vi "Array Weighted Average.vi"(4 "Reject NaN (T)":bool=TRUE, 6 "Reject Negative Weights (F)":bool, 8 "Error In":errorcluster, 9 "Weight Array":dbl[](array[numeric]), 11 "Array":dbl[](array[numeric])) -> (0 "Error Out":errorcluster, 1 "SDV (weighted)":dbl, 2 "SDV (classic)":dbl, 3 "Average Value (weighted)":dbl)   [LabVIEW 2021, in "Arrays.lvlib"]
doc: "Compute a weighted average of the input <B>Array</B> A using the provided <B>Weight Array</B> w:\n\n<A> = (Sum(w_i A_i)_{i = 1....N})/(Sum(w_i)_{i = 1....N})\n\nwhere {A_i}_{i = 1....N} is the input <B>Array</B> and {w_i}_{i = 1....N} is the <B>Weight Array</B>.\n\nIf <B>Reject Negative Weights</B> is true, only the term with w_i >= 0 are retained in both sums.\n\nIf the two arrays have different sizes, the unweighted mean of <B>Array</B> is returned.\n\nTo reject NaN values in the calculation, use the <B>Reject NaN</B> flag."
uses:
  Arrays.lvlib
  <userlib>/_OpenG.lib/array/array.llb/Filter 1D Array with Scalar (DBL)__ogtk.vi
  <vilib>/Analysis/NI_AALBase.lvlib
  <userlib>/_OpenG.lib/array/array.llb/openg_array.lvlib
  <userlib>/_OpenG.lib/array/array.llb/Delete Elements from 1D Array (DBL)__ogtk.vi
panel:
  # "see the AlliGator License on the block diagram (Ctrl+E or Window:Show Block Diagram)"
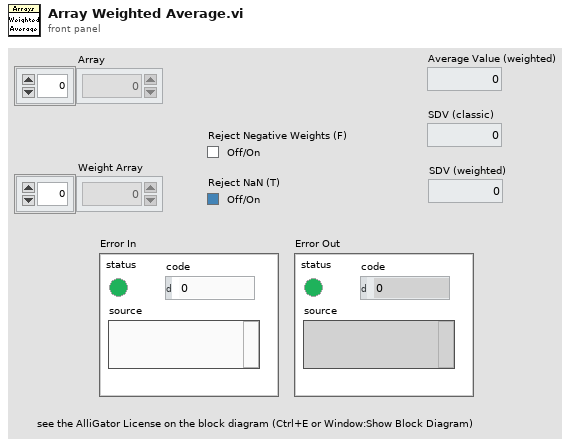
[diagram p1: front panel]
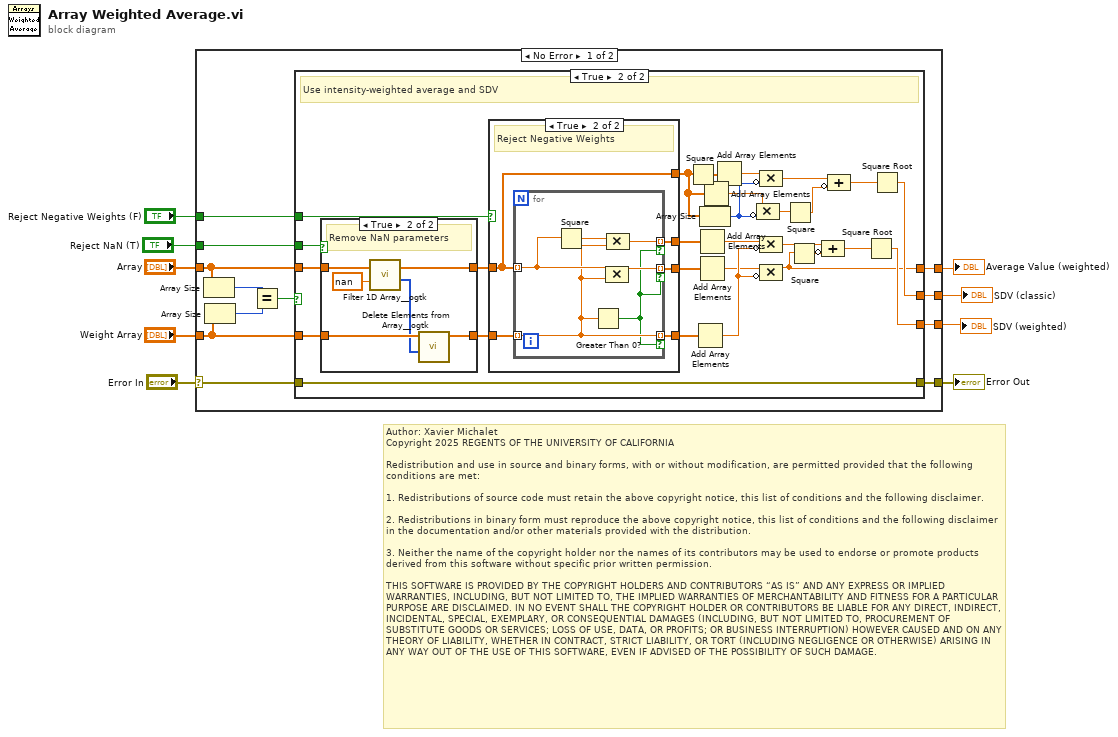
[diagram p0: block diagram]
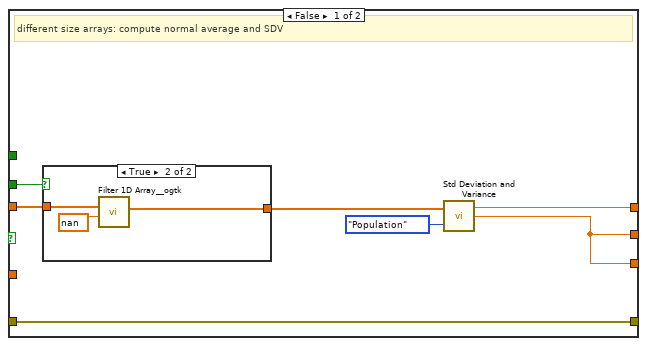
[diagram p2: hidden frame]
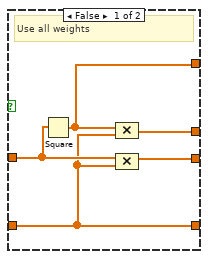
[diagram p5: hidden frame]
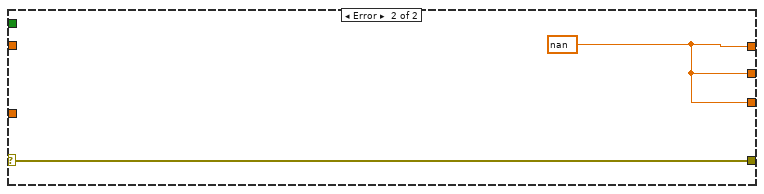
[diagram p6: hidden frame]
diagram:
  # "Author: Xavier Michalet\nCopyright 2025 REGENTS OF THE UNIVERSITY OF CALIFORNIA\n\nRedistribution and use in source and binary forms, with or without modification, are permitted provided that the following conditions are met:\n\n1. Redistributions of source code must retain the above copyright notice, this list of conditions and the following disclaimer.\n\n2. Redistributions in binary form must reproduce the above copyright notice, this list of conditions and the following disclaimer in the documentation and/or other materials provided with the distribution.\n\n3. Neither the name of the copyright holder nor the names of its contributors may be used to endorse or promote products derived from this software without specific prior written permission.\n\nTHIS SOFTWARE IS PROVIDED BY THE COPYRIGHT HOLDERS AND CONTRIBUTORS “AS IS” AND ANY EXPRESS OR IMPLIED WARRANTIES, INCLUDING, BUT NOT LIMITED TO, THE IMPLIED WARRANTIES OF MERCHANTABILITY AND FITNESS FOR A PARTICULAR PURPOSE ARE DISCLAIMED. IN NO EVENT SHALL THE COPYRIGHT HOLDER OR CONTRIBUTORS BE LIABLE FOR ANY DIRECT, INDIRECT, INCIDENTAL, SPECIAL, EXEMPLARY, OR CONSEQUENTIAL DAMAGES (INCLUDING, BUT NOT LIMITED TO, PROCUREMENT OF SUBSTITUTE GOODS OR SERVICES; LOSS OF USE, DATA, OR PROFITS; OR BUSINESS INTERRUPTION) HOWEVER CAUSED AND ON ANY THEORY OF LIABILITY, WHETHER IN CONTRACT, STRICT LIABILITY, OR TORT (INCLUDING NEGLIGENCE OR OTHERWISE) ARISING IN ANY WAY OUT OF THE USE OF THIS SOFTWARE, EVEN IF ADVISED OF THE POSSIBILITY OF SUCH DAMAGE."
  n1 = case shown="No Error" "Error In" {
    selector: "Error In" -> [w13 w86]
    tunnel: "Array" -> [w15 _]
    tunnel: [w19 w85] -> w8
    tunnel: [w12 w86] -> w6
    tunnel: "Weight Array" -> [w14 _]
    tunnel: "Reject Negative Weights (F)" -> [w18 _]
    tunnel: "Reject NaN (T)" -> [w16 _]
    tunnel: [w11 w85] -> w2
    tunnel: [w10 w85] -> w1
    frame No Error {
      n2 = Array Size(array=w15) -> (size(s)=w21:i32)
      n3 = Array Size(array=w14) -> (size(s)=w20:i32)
      n4 = Equal?(x=w21, y=w20) -> (x = y?=w17:bool)
      n5 = case shown="True" w17 {
        tunnel: [w25 w37] -> w19
        tunnel: w14 -> [_ w60]
        tunnel: w18 -> [_ w59]
        tunnel: w15 -> [w28 w58]
        tunnel: w16 -> [w27 w53]
        tunnel: w13 -> [w24 w52]
        tunnel: [w24 w52] -> w12
        tunnel: [w23 w48] -> w11
        tunnel: [w23 w39] -> w10
        frame False {
          # "different size arrays: compute normal average and SDV"
          n6 = case shown="True" w27 {
            tunnel: w28 -> [w29 w32]
            tunnel: [w29 w30] -> w26
            frame False {
            }
            frame True {
              n7 = call-poly <userlib>:"Filter 1D Array__ogtk.vi"("items to filter"=nan, "array"=w32) -> ("filtered array"=w30:dbl[])  [unwired: 4 in, 1 out]
            }
          }
          n8 = call <vilib>:"Std Deviation and Variance.vi"("X"=w26, "Weighting (Sample)"=enum16{"Sample", "Population"}."Population") -> ("mean"=w25:dbl, "standard deviation"=w23:dbl)  [unwired: 1 out]
        }
        frame True {
          # "Use intensity-weighted average and SDV"
          n9 = case shown="True" w53 {
            tunnel: w60 -> [w61 w68]
            tunnel: w58 -> [w62 w67]
            tunnel: [w62 w66] -> w57
            tunnel: [w61 w63] -> w56
            frame False {
            }
            frame True {
              # "Remove NaN parameters"
              n10 = call-poly <userlib>:"Filter 1D Array__ogtk.vi"("items to filter"=nan, "array"=w67) -> ("filtered item indices"=w64:i32[], "filtered array"=w66:dbl[])  [unwired: 4 in]
              n11 = call-poly <userlib>:"Delete Elements from Array__ogtk.vi"("indices"=w64, "array"=w68) -> ("array w/ subset deleted"=w63:dbl[])  [unwired: 8 in, 1 out]
            }
          }
          n12 = case shown="True" w59 {
            tunnel: w56 -> [w71 w78]
            tunnel: w57 -> [w72 w74]
            tunnel: [w73 w77] -> w55
            tunnel: [w71 w76] -> w54
            tunnel: [w70 w75] -> w47
            tunnel: [w69 w74] -> w34
            frame False {
              # "Use all weights"
              n13 = Square(x=w72) -> (x^2=w69:dbl[])
              n14 = Compound Arithmetic op=MULTIPLY(w69, w71) -> (w70:dbl[])
              n15 = Compound Arithmetic op=MULTIPLY(w72, w71) -> (w73:dbl[])
            }
            frame True {
              # "Reject Negative Weights"
              n16 = for {
                tunnel: w78 -> [w81] mode=indexing
                tunnel: w74 -> [w83] mode=indexing
                tunnel: [w84] -> w77 mode=indexing if=w79
                tunnel: [w81] -> w76 mode=indexing if=w79
                tunnel: [w80] -> w75 mode=indexing if=w79
                n17 = Square(x=w83) -> (x^2=w82:dbl)
                n18 = Greater Than 0?(x=w81) -> (x > 0?=w79:bool)
                n19 = Compound Arithmetic op=MULTIPLY(w83, w81) -> (w84:dbl)
                n20 = Compound Arithmetic op=MULTIPLY(w82, w81) -> (w80:dbl)
              }
            }
          }
          n21 = Square(x=w34) -> (x^2=w35:dbl[])
          n22 = Add Array Elements(numeric array=w54) -> (sum=w46:dbl)
          n23 = Add Array Elements(numeric array=w47) -> (sum=w41:dbl)
          n24 = Add Array Elements(numeric array=w55) -> (sum=w38:dbl)
          n25 = Array Size(array=w34) -> (size(s)=w43:i32)
          n26 = Add Array Elements(numeric array=w34) -> (sum=w33:dbl)
          n27 = Add Array Elements(numeric array=w35) -> (sum=w50:dbl)
          n28 = Compound Arithmetic op=MULTIPLY(w33, invert w43) -> (w42:dbl)
          n29 = Compound Arithmetic op=MULTIPLY(w50, invert w43) -> (w49:dbl)
          n30 = Compound Arithmetic op=MULTIPLY(w41, invert w46) -> (w45:dbl)
          n31 = Compound Arithmetic op=MULTIPLY(w38, invert w46) -> (w37:dbl)
          n32 = Square(x=w42) -> (x^2=w44:dbl)
          n33 = Square(x=w37) -> (x^2=w36:dbl)
          n34 = Compound Arithmetic op=ADD(w45, invert w36) -> (w40:dbl)
          n35 = Compound Arithmetic op=ADD(w49, invert w44) -> (w51:dbl)
          n36 = Square Root(x=w40) -> (sqrt(x)=w39:dbl)
          n37 = Square Root(x=w51) -> (sqrt(x)=w48:dbl)
        }
      }
    }
    frame Error {
      w85 = nan ("mean")
    }
  }
  "Average Value (weighted)" <- w8
  "Error Out" <- w6
  "SDV (classic)" <- w2
  "SDV (weighted)" <- w1
